vi "Init.vi"(8 "error in (no error)":errorcluster, 10 "Group Config":refnum<class "Group Config.lvclass">) -> (0 "error out":errorcluster, 3 "Group":refnum<class "GroupAbstract.lvclass">)   [LabVIEW 2020, in "Vecto.lvlib" / "GroupAbstract.lvclass"]
uses:
  GroupAbstract.lvclass
  Group Config/Group Config.lvclass
  Group Config/Group Config.lvclass/Group Config.ctl
  Ref.ctl
  Channel Info.ctl
  GroupAbstract.lvclass/GroupAbstract.ctl
  01584b93-a09b-41fa-a727-74251d7e872a.vi
  Vecto.lvlib
  Channel Config/Channel Config.lvclass
  Group/Group.lvclass
  StringGroup/StringGroup.lvclass
  C:/dev/lv20CE/relink/lv-vecto/Vecto/GroupAbstract/GroupAbstract.lvclass
  C:/dev/lv20CE/relink/lv-vecto/Vecto/Group/Group.lvclass
  C:/dev/lv20CE/relink/lv-vecto/Vecto/StringGroup/StringGroup.lvclass
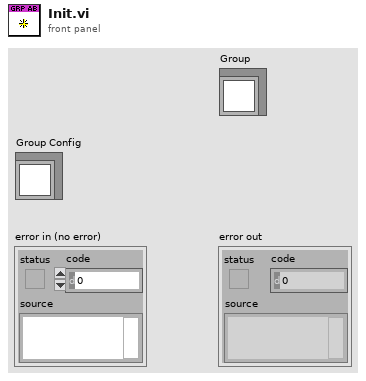
[diagram p1: front panel]
types:
  T1 = typedef "Vecto.lvlib/Channel Info.ctl" = cluster{"Name":string, "Group":string, "Owning Node":string, "Owning Task":string, "Resource":string}
  T2 = typedef "Vecto.lvlib/Group Data Type.ctl" = enum16{"Double", "String"}
  T3 = typedef "Vecto.lvlib/GroupAbstract.lvclass/Ref.ctl" = cluster{"Channel Index Map":map{string, i32}, "Channel Info":T1[]}
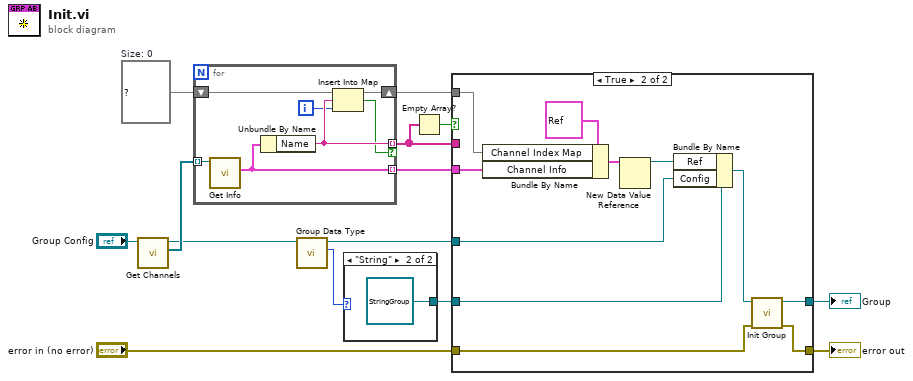
[diagram p0: block diagram]
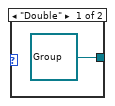
[diagram p2: hidden frame]
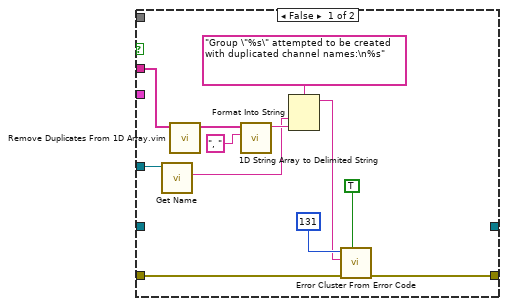
[diagram p3: hidden frame]
diagram:
  w14 = map{string, i32} {}  # Size: 0
  n1 = call "Get Channels.vi"("Group Config in"="Group Config") -> ("Channels"=w9:refnum<class "Channel Config.lvclass">[], "Group Config out"=w4:refnum<class "Group Config.lvclass">)  [unwired: 8 in, 1 out]
  n2 = for {
    tunnel: w9 -> [w16] mode=indexing
    tunnel: [w15] -> w12 mode=indexing
    shift-right: [w20] -> w13
    shift-left: w14 -> [w21]
    tunnel: [w19] -> w11 mode=indexing if=w18
    i -> [w17]
    n3 = call "Get Info.vi"("Channel Config in"=w16) -> ("Info"=w15:T1)  [unwired: 8 in, 2 out]
    n4 = Unbundle By Name(w15) -> ("Name"=w19:string)
    n5 = Insert Into Map(map in=w21, key=w19, value=w17) -> (map out=w20:map{string, i32}, key already included?=w18:bool)  [unwired: 1 out]
  }
  n6 = call "Group Data Type.vi"("Group Config in"=w4) -> ("Data Type"=w2:T2, "Group Config out"=w3:refnum<class "Group Config.lvclass">)  [unwired: 8 in, 1 out]
  n7 = case shown="\"String\"" w2 {
    tunnel: [refnum<class "Group.lvclass"> refnum ("Vecto.lvlib:Group.lvclass") refnum<class "StringGroup.lvclass"> refnum ("Vecto.lvlib:StringGroup.lvclass")] -> w1
    frame "Double" {
    }
    frame "String" {
    }
  }
  n8 = Empty Array?(array=w11) -> (empty?=w10:bool)
  n9 = case shown="True" w10 {
    tunnel: [_ w42] -> w5
    tunnel: w3 -> [w25 w36]
    tunnel: "error in (no error)" -> [w35 w40]
    tunnel: [w28 w41] -> w6
    tunnel: w13 -> [_ w43]
    tunnel: w12 -> [_ w44]
    tunnel: w11 -> [w27 _]
    tunnel: w1 -> [_ w37]
    frame False {
      n10 = call "Get Name.vi"("Group Config in"=w25) -> ("Name"=w24:string)  [unwired: 8 in, 2 out]
      n11 = call "Remove Duplicates From 1D Array.vim"("array"=w27) -> ("array with duplicates removed"=w26:string[])  [unwired: 10 in]
      n12 = call <vilib>:"1D String Array to Delimited String.vi"("delimiter"=", ", "string array"=w26) -> ("delimited string"=w30:string)  [unwired: 9 in]
      n13 = Format Into String(format string="Group \"%s\" attempted to be created with duplicated channel names:\n%s", w24, w30) -> (resulting string=w29:string)  [unwired: 2 in, 1 out]
      n14 = call <vilib>:"Error Cluster From Error Code.vi"("show call chain? (False)"=TRUE, "error in (no error)"=w35, "error message (\"\")"=w29, "error code (0)"=131) -> ("error out"=w28:errorcluster)  [unwired: 5 in]
    }
    frame True {
      n15 = Bundle By Name(cluster=T3 {"Channel Index Map"={}, "Channel Info"=[]} ("Ref"), "Channel Index Map"=w43, "Channel Info"=w44) -> (w45:T3)
      n16 = New Data Value Reference(data value=w45) -> (data value reference=w38:refnum<data-value>)  [unwired: 1 in, 1 out]
      n17 = Bundle By Name(cluster=w37, "Ref"=w38, "Config"=w36) -> (w39:refnum<class "GroupAbstract.lvclass">)
      n18 = call-dynamic "Init Group.vi"("error in (no error)"=w40, "GroupAbstract in"=w39) -> ("error out"=w41:errorcluster, "GroupAbstract out"=w42:refnum<class "GroupAbstract.lvclass">)  [unwired: 8 in]
    }
  }
  "error out" <- w6
  "Group" <- w5
